vi "Channel_WriteLogWfm.vi"(7 "t0":timestamp, 8 "error in (no error)":errorcluster, 9 "Group Name":string, 10 "tdms file":refnum<k34>, 11 "Channel in":refnum<class "Channel.lvclass">) -> (0 "error out":errorcluster, 2 "tdms file out":refnum<k34>, 3 "Channel out":refnum<class "Channel.lvclass">)   [LabVIEW 2023, in "Channel.lvclass"]
doc: "Write the waveform channel data to file whilst downsampling."
uses:
  Channel.lvclass
  Channel.lvclass/Channel.ctl
  <vilib>/NI VeriStand/Custom Device Waveform API/Waveform Session.lvclass/Waveform Session.ctl
  <vilib>/NI VeriStand/Custom Device Waveform API/Single Waveform Read (DBL)/Single Waveform Read (DBL).lvclass/Single Waveform Read (DBL).ctl
  <vilib>/NI VeriStand/Custom Device Waveform API/Internal Comm Classes/WPL Comm/WPL Comm (1D DBL)/WPL Comm (1D DBL).lvclass/WPL Comm (1D DBL).ctl
  <vilib>/NI VeriStand/Custom Device Waveform API/Single Waveform Read (DBL)/NI VeriStand - Read Single Waveform (DBL).vi
  <vilib>/NI VeriStand/Custom Device Waveform API/Internal Comm Classes/WPL Comm/WPL Comm (1D DBL)/Comm_read 1d dbl.vi
  <vilib>/NI VeriStand/Custom Device Waveform API/Check Opened.vi
  <vilib>/NI VeriStand/Custom Device Waveform API/Internal Comm Classes/WPL Comm/Convert Q Error to Shutdown Error.vi
  <vilib>/NI VeriStand/Custom Device Waveform API/Single Waveform Read (DBL)/Single Waveform Read (DBL).lvclass
  C:/Program Files/National Instruments/LabVIEW 2024/vi.lib/NI VeriStand/Custom Device Waveform API/Waveform Session.lvclass
  <vilib>/Utility/error.llb/Error Cluster From Error Code.vi
  <vilib>/Analysis/2dsp.llb/Decimate (continuous, DBL).vi
  <vilib>/Analysis/NI_AALPro.lvlib
  <vilib>/NI VeriStand/Custom Device Waveform API/NI_VS Custom Device Waveform API.lvlib
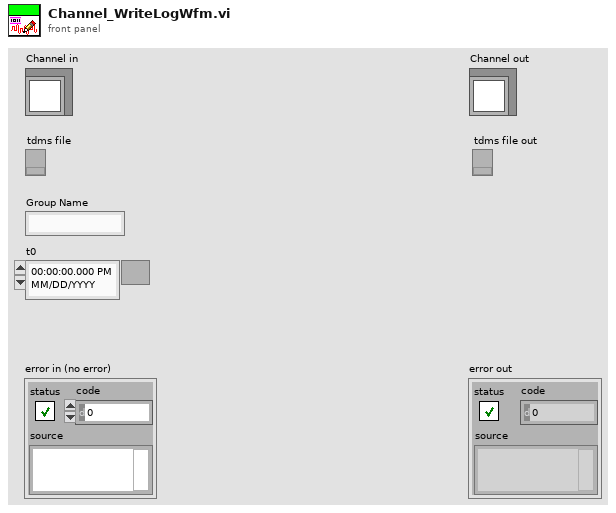
[diagram p1: front panel]
types:
  T1 = typedef "NI_VS Custom Device Waveform API.lvlib/Waveform properties.ctl" = cluster{"Data reference":T2, "t0 at start":timestamp, "dt":dbl, "offset from start (samples)":u64}
  T2 = typedef "Custom Device API.lvlib/Waveform Data Reference.ctl" = i32
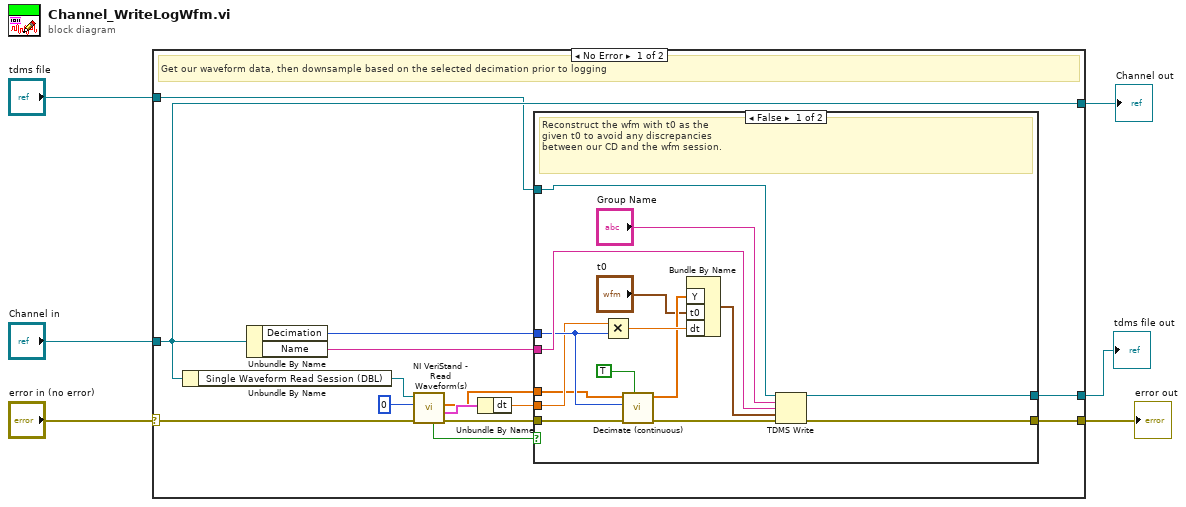
[diagram p0: block diagram]
diagram:
  n1 = case shown="No Error" "error in (no error)" {
    selector: "error in (no error)" -> [w11 w40]
    tunnel: [w10 w40] -> w5
    tunnel: [w12 w39] -> w3
    tunnel: "Channel in" -> [w12 w39]
    tunnel: [w8 w38] -> w2
    tunnel: "tdms file" -> [w7 w38]
    frame No Error {
      # "Get our waveform data, then downsample based on the selected decimation prior to logging"
      n2 = Unbundle By Name(w12) -> ("Single Waveform Read Session (DBL)"=w13:refnum<class "Single Waveform Read (DBL).lvclass">)
      n3 = Unbundle By Name(w12) -> ("Decimation"=w9:i32, "Name"=w20:string)
      n4 = call-poly <vilib>:"NI VeriStand - Read Waveform(s).vi"("error in (no error)"=w11, "timeout in ms (-1)"=0, "Single Waveform Read Session (DBL) in"=w13) -> ("error out"=w14:errorcluster, "Properties"=w18:T1, "Data"=w16:dbl[], "timed out?"=w15:bool)  [unwired: 4 in, 1 out]
      n5 = Unbundle By Name(w18) -> ("dt"=w19:dbl)
      n6 = case shown="False" w15 {
        tunnel: w20 -> [w35 _]
        tunnel: [w34 w37] -> w10
        tunnel: w19 -> [w28 _]
        tunnel: w9 -> [w29 _]
        tunnel: w14 -> [w26 w37]
        tunnel: w16 -> [w27 _]
        tunnel: w7 -> [w22 w36]
        tunnel: [w21 w36] -> w8
        frame False {
          # "Reconstruct the wfm with t0 as the\ngiven t0 to avoid any discrepancies\nbetween our CD and the wfm session."
          n7 = Multiply(x=w28, y=w29) -> (x*y=w33:dbl)
          n8 = call-poly <vilib>:"Decimate (continuous).vi"("reset"=TRUE ("averaging"), "error in (no error)"=w26, "decimating factor"=w29, "X"=w27) -> ("error out"=w25:errorcluster, "Decimated Array"=w31:dbl[])  [unwired: 6 in]
          n9 = Bundle By Name("Y"=w31, "t0"="t0", "dt"=w33) -> (w32:waveform(dbl))  [unwired: 1 in]
          n10 = TDMS Write(0:w22, 5:"Group Name", 7:w35, 9:w32, 11:w25) -> (4:w21:refnum<k34>, 15:w34:errorcluster)  [unwired: 1 in, 2 out]
        }
        frame True {
          # "No data was captured, possibly the wfm is not running or we're running faster than the wfm is producing data."
        }
      }
    }
    frame Error {
    }
  }
  "error out" <- w5
  "Channel out" <- w3
  "tdms file out" <- w2
